vi "Dialog Window Setup.vi"(7 "Action":enum16{"Pre-Populate", "Post-Populate"}(ring), 8 "error in":errorcluster, 10 "Dialog VI Ref In [Parent]":refnum<vi>, 11 "Align-to Window Ref":refnum<vi>) -> (0 "error out":errorcluster, 2 "Dialog VI Ref Out":refnum<vi>)   [LabVIEW 2023]
doc: "Pre-populate mode opens the FP in a hidden state, aligns the window to the calling VI (if ref wired in), sets pane origina of all panes, and sets the behavior of the reightmost splitter, which divides the viewed area of the FP from the developer's area.\n\nAfter running prepopulate, you can continue to set up other FP features before running this VI in post-poluate mode, which maes the FP visible and active. \n\nAlign Dialog to a scripted block diagram window, prepare dialog FP (resizing) and open it for view. If Dialog ref is not passesd in it's assumed to be the parent of this VI."
uses:
  <userlib>/_OpenG.lib/appcontrol/appcontrol.llb/openg_application_control.lvlib
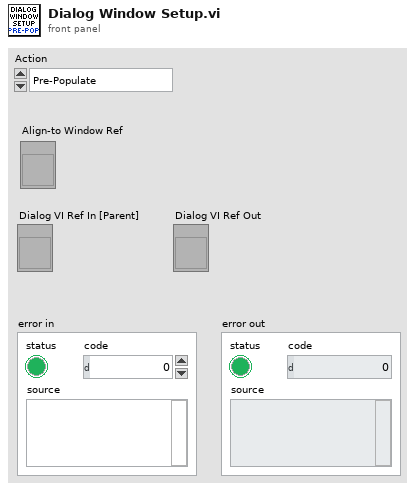
[diagram p1: front panel]
types:
  T1 = enum32{"Invalid", "Standard", "Closed", "Hidden", "Minimized", "Maximized"}
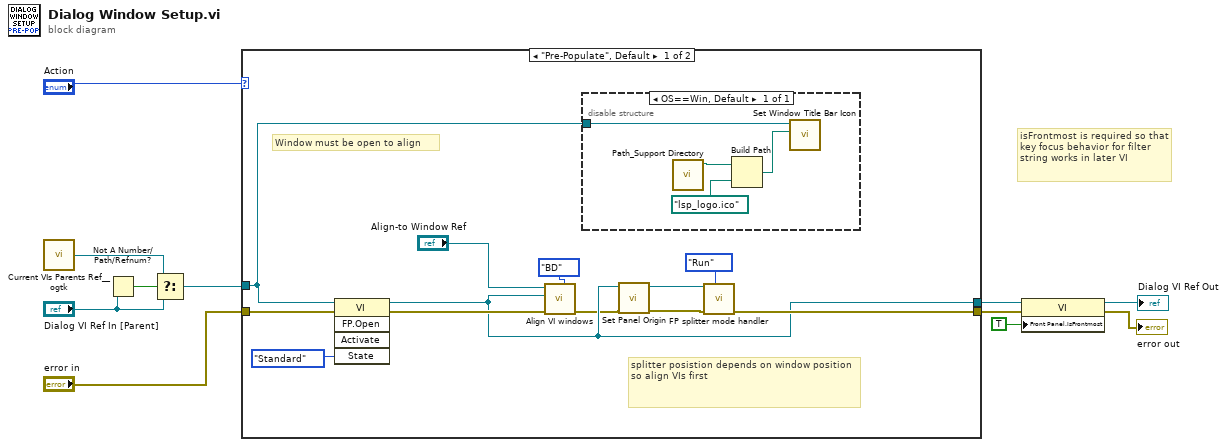
[diagram p0: block diagram]
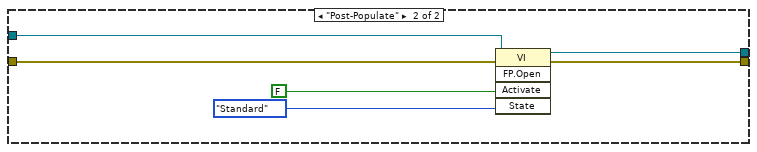
[diagram p2: hidden frame]
diagram:
  # "isFrontmost is required so that key focus behavior for filter string works in later VI"
  n1 = call <userlib>:"Current VIs Parents Ref__ogtk.vi"() -> ("Calling VI's Reference"=w10:refnum<vi>)  [unwired: 2 in]
  n2 = Not A Number/Path/Refnum?(number/path/refnum="Dialog VI Ref In [Parent]") -> (NaN/Path/Refnum?=w7:bool)
  n3 = Select(t=w10, s=w7, f="Dialog VI Ref In [Parent]") -> (s? t:f=w9:refnum<vi>)
  n4 = case shown="\"Pre-Populate\", Default" "Action" {
    tunnel: [w16 w31] -> w3
    tunnel: [w20 w33] -> w5
    tunnel: w9 -> [w12 w28]
    tunnel: "error in" -> [w22 w29]
    frame "Pre-Populate", Default {
      # "splitter posistion depends on window position so align VIs first"
      # "Window must be open to align"
      n5 = invoke class="VI" method="FP.Open"(reference=w12, error in=w22, "State"=T1."Standard") -> (reference out=w16:refnum<vi>, error out=w19:errorcluster)  [unwired: 2 in, 3 out]
      n6 = call "Align VI windows.vi"("Align to"=enum16{"FP", "BD"}."BD", "error in"=w19, "VI to Move Ref"=w16, "Stationary VI Ref"="Align-to Window Ref") -> ("error out"=w15:errorcluster)  [unwired: 7 in]
      n7 = disable-structure shown="OS==Win, Default" {
        disable-tunnel: w12 -> [w27]
        frame condition #0 (active) {
          n8 = call "Path_Support Directory.vi"() -> ("Support Directory"=w24:path)  [unwired: 11 in]
          n9 = Build Path(base path=w24, name or relative path=path "lsp_logo.ico" ("ICO Icon")) -> (appended path=w25:path)
          n10 = call "Set Window Title Bar Icon.vi"("ICO Icon"=w25, "VIRef"=w27) -> ()  [unwired: 9 in, 1 out]
        }
      }
      n11 = call "Set Panel Origin.vi"("error in"=w15, "VI Ref In"=w16) -> ("error out"=w13:errorcluster, "VI Ref Out"=w14:refnum<vi>)  [unwired: 8 in]
      n12 = call "FP splitter mode handler.vi"("Mode"=enum16{"Run", "Development"}."Run", "error in"=w13, "VI Ref In"=w14) -> ("error out"=w20:errorcluster)  [unwired: 7 in, 1 out]
    }
    frame "Post-Populate" {
      n13 = invoke class="VI" method="FP.Open"(reference=w28, error in=w29, "Activate"=FALSE ("Activate?"), "State"=T1."Standard") -> (reference out=w31:refnum<vi>, error out=w33:errorcluster)  [unwired: 1 in, 3 out]
    }
  }
  n14 = property class="VI"(reference=w3, error in=w5, "Front Panel.IsFrontmost"=TRUE ("Front Panel Window:Is Frontmost")) -> (reference out=→"Dialog VI Ref Out":refnum<vi>, error out=→"error out":errorcluster)
